vi "GL Set Operation Mode.vi"(5 "LimitWarning?":bool=TRUE, 6 "position cts (abs/rel)":i32, 7 "Position Mode (Absolute)":T2(ring), 8 "error in (no error)":errorcluster, 9 "Start Now?":bool, 10 "Axis":T1 items=["Axis 1", "Axis 2", "Axis 3", "Axis 4", "Axis 5", "Axis 6", "Axis 7", "Axis 8"], 11 "Galil.IGalil":refnum<k7>) -> (0 "error out":errorcluster, 2 "Axis Out Output":T1 items=["Axis 1", "Axis 2", "Axis 3", "Axis 4", "Axis 5", "Axis 6", "Axis 7", "Axis 8"], 3 "Galil Out":refnum<k7>)   [LabVIEW 2022 SP3]
doc: "Sets the operation mode for an axis or vector space."
uses:
  GL Axis Control.ctl
  Command Menu.ctl
panel:
  out "Response:":string
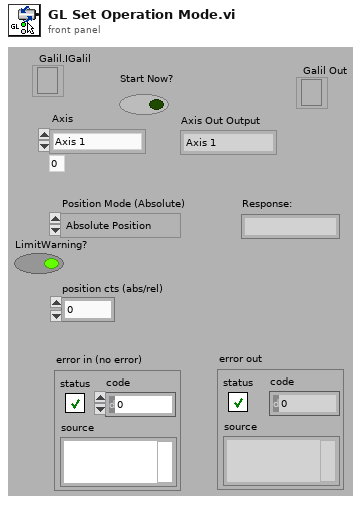
[diagram p1: front panel]
types:
  T1 = typedef "GL Axis Control.ctl" = u16
  T2 = enum16{"Absolute Position", "Relative Position", "Velocity", "Relative to Cap Pos", "Modulus Position", "Absolute Contouring", "Relative Contouring"}
  T3 = typedef "Command Menu.ctl" = enum16{"CommandPassThrough", "Abort Motion", "Define Pos", "Velocity", "Acceleration", "Deceleration", "Position Rel", "Postion Abs", "Begin Move", "After Move", "Home", "KI", "KD", "KP", "IL", "Config I/O", "Set Bit", "Clear Bit", "Motor Off", "Moto On", "Status", "Execute", "Halt Execute", "HX Status", "Tell Velocity", "Check Motion", "BreakPoint", "Tell Position", "Current Code Line", "Tell Switches", "OC Force On", "OC Off", "Pos Soft Limit", "Rev Soft Limit"}
  T4 = cluster{"HomeStatus":bool, "ReverseLimit?":bool, "ForwardLimit?":bool, "LimitHit?":bool, "MotorOff?":bool, "Motion?":bool}
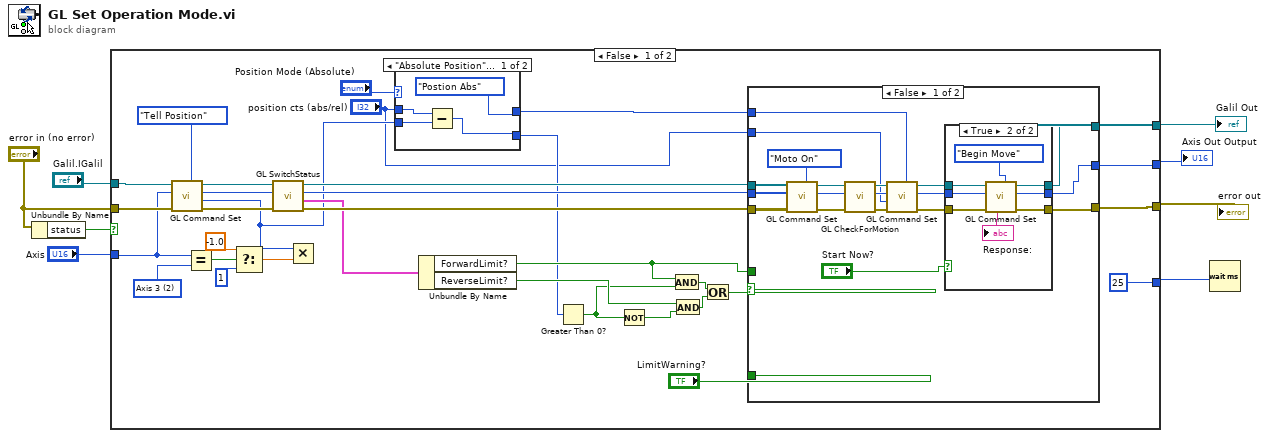
[diagram p0: block diagram]
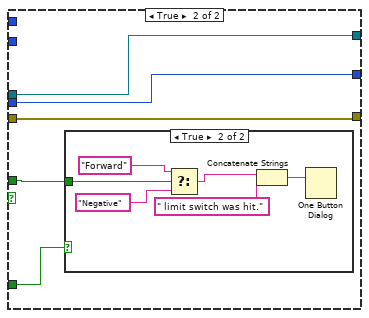
[diagram p3: hidden frame]
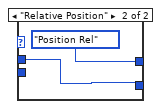
[diagram p5: hidden frame]
diagram:
  n1 = Unbundle By Name("error in (no error)") -> ("status"=w6:bool)
  n2 = case shown="False" w6 {
    tunnel: "error in (no error)" -> [w32 w91]
    tunnel: [w10 w91] -> w7
    tunnel: "Galil.IGalil" -> [w36 w90]
    tunnel: [w9 w90] -> w4
    tunnel: [w11 w89] -> w3
    tunnel: "Axis" -> [w18 w89]
    tunnel: [25 _] -> w1
    frame False {
      w17 = T1 2 items=["Axis 1", "Axis 2", "Axis 3", "Axis 4", "Axis 5", "Axis 6", "Axis 7", "Axis 8"] ("Axis")
      n3 = call "GL Command Set.vi"("Command"=Command_Menu."Tell Position", "error in (no error)"=w32, "Axis"=w18, "Galil.IGalil"=w36) -> ("error out"=w31:errorcluster, "Response#"=w13:i32, "Axis Out"=w33:T1, "ref out"=w35:refnum<k7>)  [unwired: 3 in, 1 out]
      n4 = Equal?(x=w18, y=w17) -> (x = y?=w16:bool)
      n5 = Select(t=-1.0, s=w16, f=1) -> (s? t:f=w20:dbl)
      n6 = call "GL SwitchStatus.vi"("error in (no error)"=w31, "Axis"=w33, "Galil.IGalil"=w35) -> ("error out"=w40:errorcluster, "TS Status"=w37:T4, "Axis Out"=w38:T1, "ref out"=w39:refnum<k7>)  [unwired: 3 in]
      n7 = Multiply(x=w13, y=w20) -> ()  [unwired: 1 out]
      n8 = case shown="\"Absolute Position\", Default" "Position Mode (Absolute)" {
        tunnel: w13 -> [w84 _]
        tunnel: "position cts (abs/rel)" -> [w85 w88]
        tunnel: [w86 w88] -> w14
        tunnel: [Command_Menu."Postion Abs" ("Command") Command_Menu."Position Rel" ("Command")] -> w15
        frame "Absolute Position", Default {
          n9 = Subtract(x=w85, y=w84) -> (x-y=w86:i32)
        }
        frame "Relative Position" {
        }
      }
      n10 = Unbundle By Name(w37) -> ("ForwardLimit?"=w26:bool, "ReverseLimit?"=w27:bool)
      n11 = Greater Than 0?(x=w14) -> (x > 0?=w19:bool)
      n12 = Not(x=w19) -> (.not. x?=w28:bool)
      n13 = And(x=w26, y=w19) -> (x .and. y?=w29:bool)
      n14 = And(x=w27, y=w28) -> (x .and. y?=w30:bool)
      n15 = Or(x=w29, y=w30) -> (x .or. y?=w23:bool)
      n16 = case shown="False" w23 {
        tunnel: [w45 w75] -> w10
        tunnel: [w46 w74] -> w9
        tunnel: w40 -> [w59 w75]
        tunnel: w39 -> [w60 w74]
        tunnel: w38 -> [w42 w76]
        tunnel: [w43 w76] -> w11
        tunnel: w26 -> [_ w73]
        tunnel: "LimitWarning?" -> [_ w72]
        tunnel: w15 -> [w51 _]
        tunnel: "position cts (abs/rel)" -> [w50 _]
        frame False {
          n17 = call "GL Command Set.vi"("Command"=Command_Menu."Moto On", "error in (no error)"=w59, "Axis"=w42, "Galil.IGalil"=w60) -> ("error out"=w58:errorcluster, "Axis Out"=w55:T1, "ref out"=w57:refnum<k7>)  [unwired: 3 in, 2 out]
          n18 = call "GL CheckForMotion.vi"("error in"=w58, "Axis"=w55, "Refnum in"=w57) -> ("error out"=w52:errorcluster, "Axis out"=w53:T1, "Refnum out"=w54:refnum<k7>)  [unwired: 6 in]
          n19 = call "GL Command Set.vi"("Command"=w51, "error in (no error)"=w52, "Value"=w50, "Axis"=w53, "Galil.IGalil"=w54) -> ("error out"=w48:errorcluster, "Axis Out"=w47:T1, "ref out"=w49:refnum<k7>)  [unwired: 2 in, 2 out]
          n20 = case shown="True" "Start Now?" {
            tunnel: w49 -> [w63 w71]
            tunnel: w48 -> [w61 w70]
            tunnel: w47 -> [w62 w69]
            tunnel: [w62 w67] -> w43
            tunnel: [w63 w66] -> w46
            tunnel: [w61 w65] -> w45
            frame False {
            }
            frame True {
              n21 = call "GL Command Set.vi"("Command"=Command_Menu."Begin Move", "error in (no error)"=w70, "Axis"=w69, "Galil.IGalil"=w71) -> ("error out"=w65:errorcluster, "Axis Out"=w67:T1, "ref out"=w66:refnum<k7>, "Response: text"=→"Response:":string)  [unwired: 3 in, 1 out]
            }
          }
        }
        frame True {
          n22 = case shown="True" w72 {
            tunnel: w73 -> [_ w82]
            frame False {
            }
            frame True {
              n23 = Select(t="Forward", s=w82, f="Negative") -> (s? t:f=w80:string)
              n24 = Concatenate Strings(w80, " limit switch was hit." ("message")) -> (w77:string)
              n25 = One Button Dialog(message=w77) -> ()  [unwired: 1 in, 1 out]
            }
          }
        }
      }
    }
    frame True {
    }
  }
  "error out" <- w7
  "Galil Out" <- w4
  "Axis Out Output" <- w3
  n26 = Wait (ms)(milliseconds to wait=w1) -> ()  [unwired: 1 out]
